vi "Get Cell Values.vi"(7 "Sheet Name":string, 8 "error in":errorcluster, 10 "Cell Addresses":string="A1:B1", 11 "SpreadsheetDoc in":refnum<k24>) -> (0 "error out":errorcluster, 1 "Types":T1[][](array[typedef]), 2 "Cell Values":T2(array[cluster]) {"Time Stamp" format="%<%x %.3X>T"}, 3 "SpreadsheetDoc out":refnum<k24>)   [LabVIEW 2019, in "Open Xml.lvlib"]
uses:
  Open Xml.lvlib
  D:/git/Open-Xml-LabVIEW/Source/DocumentFormat.OpenXml.dll
  DocumentFormat.OpenXml.dll
  Cell DataType.ctl
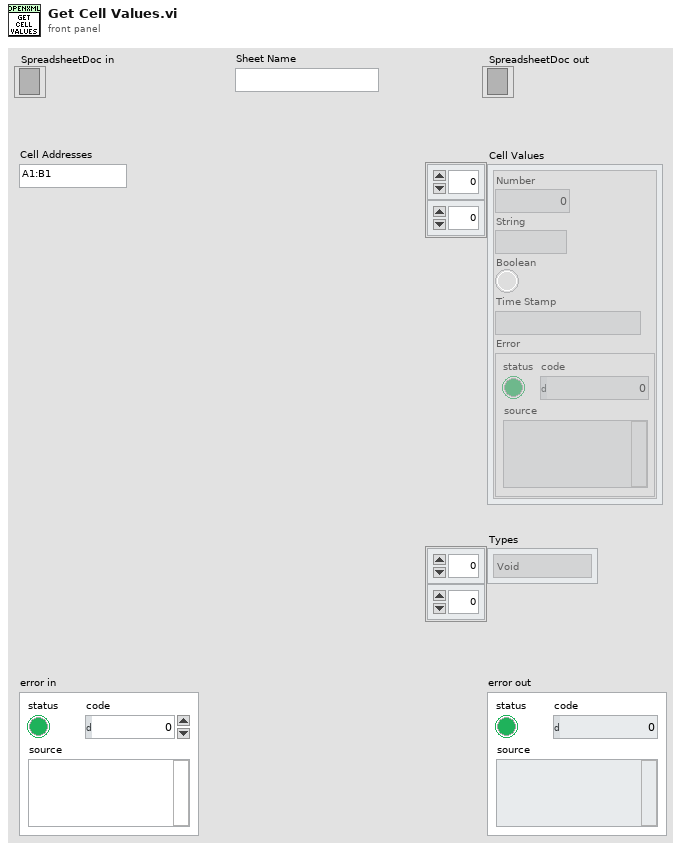
[diagram p1: front panel]
types:
  T1 = typedef "Open Xml.lvlib/Cell DataType.ctl" = enum16{"Void", "Boolean", "Number", "Error", "SharedString", "String", "InlineString", "Date"}
  T2 = cluster{"Number":dbl, "String":string, "Boolean":bool, "Time Stamp":timestamp, "Error":errorcluster}[][]
  T3 = cluster{"Number":dbl, "String":string, "Boolean":bool, "Time Stamp":timestamp, "Error":errorcluster}
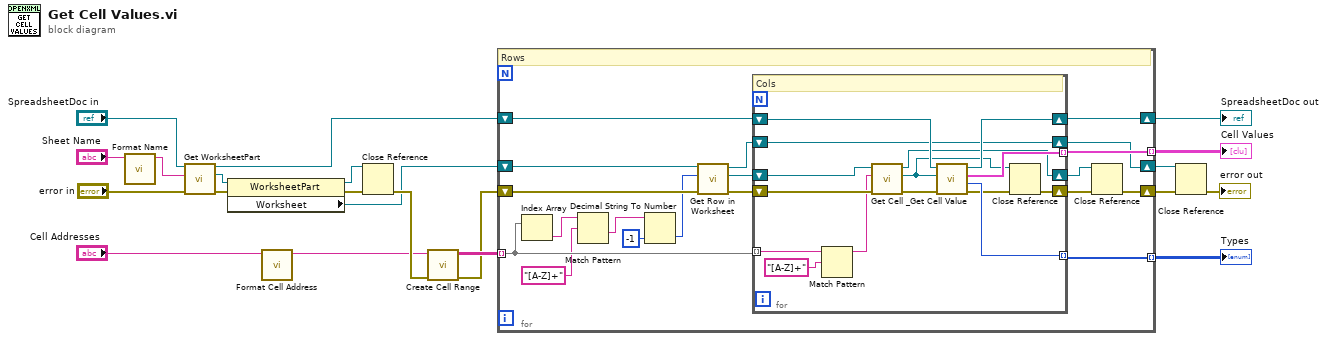
[diagram p0: block diagram]
diagram:
  n1 = call "Format Name.vi"("Sheet Name"="Sheet Name") -> ("Formatted Sheet Name"=w1:string)  [unwired: 10 in]
  n2 = call "Get WorksheetPart.vi"("error in"="error in", "Sheet Name"=w1, "SpreadsheetDoc in"="SpreadsheetDoc in") -> ("error out"=w8:errorcluster, "WorksheetPart"=w7:refnum<k24>, "SpreadsheetDoc out"=w15:refnum<k24>)  [unwired: 5 in, 1 out]
  n3 = property class="WorksheetPart"(reference=w7, error in=w8) -> (reference out=w4:refnum<k24>, error out=w6:errorcluster, "Worksheet"=w3:refnum<k24>)
  n4 = call "Format Cell Address.vi"("Cell Address"="Cell Addresses") -> ("Formatted Cell Address"=w2:string)  [unwired: 10 in]
  n5 = Close Reference(reference=w4, error in (no error)=w6) -> (error out=w5:errorcluster)
  n6 = call "Create Cell Range.vi"("error in"=w5, "Cell Range"=w2) -> ("error out"=w11:errorcluster, "Cell Range"=w18:string[][])  [unwired: 8 in]
  n7 = for {
    tunnel: w18 -> [w30] mode=indexing
    tunnel: [w37] -> w14 mode=indexing
    tunnel: [w36] -> w13 mode=indexing
    shift-right: [w39] -> w19
    shift-left: w15 -> [w38]
    shift-right: [w23] -> w20
    shift-left: w11 -> [w34]
    shift-right: [w35] -> w12
    shift-left: w3 -> [w32]
    # "Rows"
    n8 = Index Array(array=w30) -> (element=w29:string)  [unwired: 1 in]
    n9 = Match Pattern(string=w29, regular expression="[A-Z]+") -> (after substring=w26:string)  [unwired: 1 in, 3 out]
    n10 = Decimal String To Number(string=w26, default (0L)=-1 ("default (0 I32)")) -> (number=w25:i32)  [unwired: 1 in, 1 out]
    n11 = call "Get Row in Worksheet.vi"("error in"=w34, "RowIndex"=w25, "Worksheet in"=w32) -> ("error out"=w33:errorcluster, "Row out"=w24:refnum<k24>, "Worksheet out"=w31:refnum<k24>)  [unwired: 6 in]
    n12 = for {
      tunnel: [w50] -> w37 mode=indexing
      tunnel: [w49] -> w36 mode=indexing
      shift-right: [w53] -> w40
      shift-left: w33 -> [w54]
      shift-right: [w51] -> w39
      shift-left: w38 -> [w52]
      tunnel: w30 -> [w44] mode=indexing
      shift-right: [w41] -> w22
      shift-left: w24 -> [w42]
      shift-right: [w43] -> w35
      shift-left: w31 -> [w43]
      # "Cols"
      n13 = Match Pattern(string=w44, regular expression="[A-Z]+") -> ()  [unwired: 1 in, 4 out]
      n14 = call "Get Cell.vi"("error in"=w54, "Cell Address"=w44, "Row in"=w42) -> ("error out"=w48:errorcluster, "Cell"=w46:refnum<k24>, "Row out"=w41:refnum<k24>)  [unwired: 6 in]
      n15 = call "_Get Cell Value.vi"("error in"=w48, "Cell"=w46, "SpreadsheetDoc in"=w52) -> ("error out"=w47:errorcluster, "Type"=w49:T1, "Cell Value"=w50:T3, "SpreadsheetDocument out"=w51:refnum<k24>)  [unwired: 5 in]
      n16 = Close Reference(reference=w46, error in (no error)=w47) -> (error out=w53:errorcluster)
    }
    n17 = Close Reference(reference=w22, error in (no error)=w40) -> (error out=w23:errorcluster)
  }
  "SpreadsheetDoc out" <- w19
  "Cell Values" <- w14
  "Types" <- w13
  n18 = Close Reference(reference=w12, error in (no error)=w20) -> (error out=→"error out":errorcluster)
